vi "InsertRamp.vi"(8 "error in (no error)":errorcluster, 11 "Pulseblaster in":refnum<class "Pulseblaster.lvclass">) -> (0 "error out":errorcluster, 3 "Pulseblaster out":refnum<class "Pulseblaster.lvclass">)   [LabVIEW 2012, in "Pulseblaster.lvclass"]
uses:
  Pulseblaster.lvclass
  PulseBlaster.lvlib
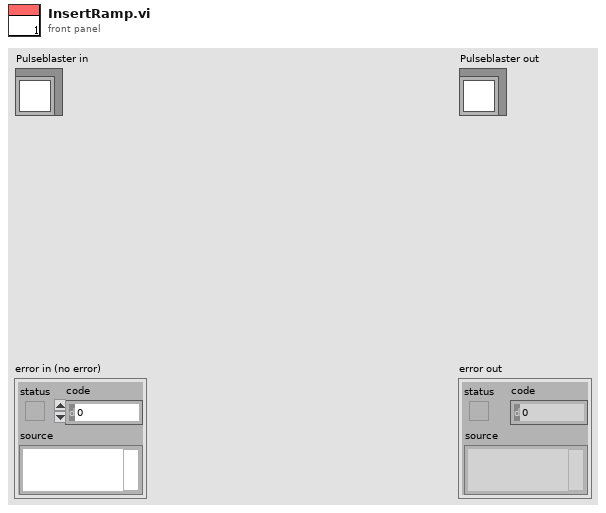
[diagram p1: front panel]
types:
  T1 = cluster{"Output Bits":u32, "Data Field":u32, "OP Code":u8, "Delay Count":u32}[]
  T2 = cluster{"Ramp Index":i32, "Ramp Time":dbl, "Number of Steps":i32}[]
  T3 = cluster{"Output Bits":u32, "Data Field":u32, "OP Code":u8, "Delay Count":u64}[]
  T4 = cluster{"Output Bits":u32, "Data Field":u32, "OP Code":u8, "Delay Count":u64}
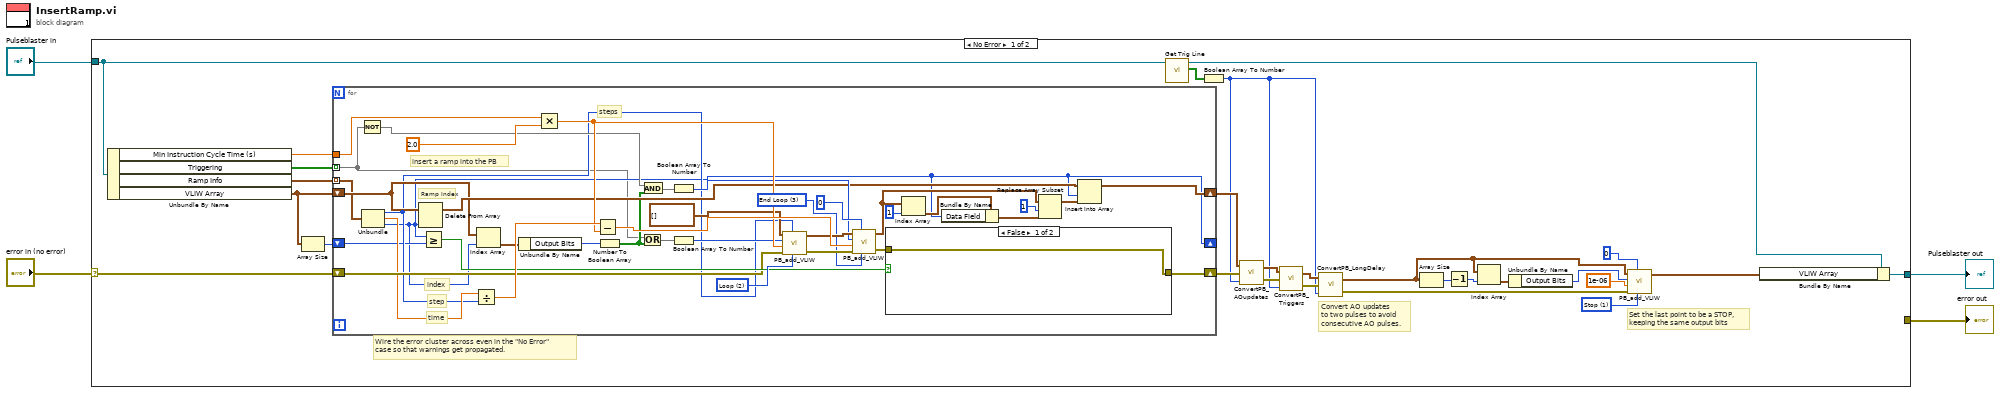
[diagram p0: block diagram]
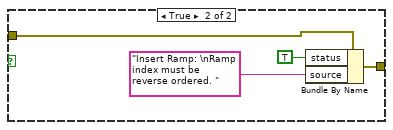
[diagram p2: hidden frame]
diagram:
  n1 = case shown="No Error" "error in (no error)" {
    selector: "error in (no error)" -> [w27 w76]
    tunnel: [_ w76] -> w3
    tunnel: [w25 w75] -> w1
    tunnel: "Pulseblaster in" -> [w26 w75]
    frame No Error {
      w14 = u8 1 items=["Continue", "Stop", "Loop", "End Loop", "Jump", "Return", "Go To", "Long Delay"] ("OP code")
      # "Convert AO updates\nto two pulses to avoid\nconsecutive AO pulses."
      # "Set the last point to be a STOP,\nkeeping the same output bits"
      # "Wire the error cluster across even in the \"No Error\"\ncase so that warnings get propagated."
      n2 = Unbundle By Name(w26) -> ("Min Instruction Cycle Time (s)"=w30:dbl, "Triggering"=w5:bool[][], "Ramp Info"=w29:T2, "VLIW Array"=w28:T3)
      n3 = Array Size(array=w28) -> (size(s)=w31:i32)
      n4 = for {
        tunnel: w29 -> [w38] mode=indexing
        shift-right: [w41] -> w11
        shift-left: w27 -> [w42]
        shift-right: [w39] -> w10
        shift-left: w28 -> [w40]
        shift-right: [w34] -> _
        shift-left: w31 -> [w35]
        tunnel: w30 -> [w33]
        tunnel: w5 -> [w32] mode=indexing
        w60 = u8 3 items=["Continue", "Stop", "Loop", "End Loop", "Jump", "Return", "Go To", "Long Delay"] ("OP code")
        w63 = u8 2 items=["Continue", "Stop", "Loop", "End Loop", "Jump", "Return", "Go To", "Long Delay"] ("OP code")
        # "steps"
        # "step"
        # "time"
        # "index"
        # "insert a ramp into the PB"
        # "Ramp Index"
        n5 = Not(x=w32) -> (.not. x?=w45:bool[])
        n6 = Unbundle(w38) -> ("Ramp Index"=w36:i32, "Ramp Time"=w37:dbl, "Number of Steps"=w34:i32)
        n7 = Delete From Array(array=w40, index=w34) -> (array with subset deleted=w49:T3)  [unwired: 1 in, 1 out]
        n8 = Greater Or Equal?(x=w34, y=w35) -> (x >= y?=w44:bool)
        n9 = Divide(x=w37, y=w36) -> (x/y=w69:dbl)
        n10 = Index Array(array=w40, index=w34) -> (element=w65:T4)
        n11 = Unbundle By Name(w65) -> ("Output Bits"=w50:u32)
        n12 = Multiply(x=w33, y=2.0) -> (x*y=w66:dbl)
        n13 = Subtract(x=w69, y=w66) -> (x-y=w68:dbl)
        n14 = Number To Boolean Array(number=w50) -> (Boolean array=w46:bool[])
        n15 = Or(x=w32, y=w46) -> (x .or. y?=w48:bool[])
        n16 = And(x=w45, y=w46) -> (x .and. y?=w47:bool[])
        n17 = Boolean Array To Number(Boolean array=w47) -> (number=w58:u32)
        n18 = Boolean Array To Number(Boolean array=w48) -> (number=w64:u32)
        n19 = call "PB_add_VLIW.vi"("VLIW Array In"=T1 [], "Data Field"=w36, "Digital Bits"=w64, "Delay"=w66, "OP code"=w63, "error in (no error)"=w42) -> ("VLIW Array Out"=w62:T3, "error out"=w61:errorcluster)  [unwired: 1 out]
        n20 = call "PB_add_VLIW.vi"("VLIW Array In"=w62, "Data Field"=u32 0, "Digital Bits"=w58, "Delay"=w68, "OP code"=w60, "error in (no error)"=w61) -> ("VLIW Array Out"=w51:T3, "error out"=w43:errorcluster)  [unwired: 1 out]
        n21 = case shown="False" w44 {
          tunnel: [w70 w72] -> w41
          tunnel: w43 -> [w70 w71]
          frame False {
          }
          frame True {
            n22 = Bundle By Name(cluster=w71, "status"=TRUE, "source"="Insert Ramp: \nRamp index must be reverse ordered. ") -> (w72:errorcluster)
          }
        }
        n23 = Index Array(array=w51, index=1 ("Index")) -> (element=w55:T4)
        n24 = Bundle By Name(cluster=w55, "Data Field"=w34) -> (w54:T4)
        n25 = Replace Array Subset(array=w51, new element=w54, index=1) -> (w52:T3)
        n26 = Insert Into Array(array=w49, index=w34, new element=w52) -> (w39:T3)
      }
      n27 = call-dynamic "Get Trig Line.vi"("Master Device in"=w26) -> ("Full Trigger Line"=w7:bool[], "Master Device out"=w8:refnum<class "Pulseblaster.lvclass">)  [unwired: 8 in, 1 out]
      n28 = Boolean Array To Number(Boolean array=w7) -> (number=w6:u32)
      n29 = call "ConvertPB_AOupdates.vi"("Full trigger mask"=w6, "error in (no error)"=w11, "PB VLIW Array in"=w10) -> ("error out"=w21:errorcluster, "PB VLIW Array out"=w20:T3)
      n30 = call "ConvertPB_Triggers.vi"("Full trigger mask"=w6, "error in (no error)"=w21, "PB VLIW Array in"=w20) -> ("error out"=w24:errorcluster, "PB VLIW Array out"=w22:T3)
      n31 = call "ConvertPB_LongDelay.vi"("Full trigger mask"=w6, "error in (no error)"=w24, "PB VLIW Array in"=w22) -> ("error out"=w12:errorcluster, "PB VLIW Array out"=w23:T3)
      n32 = Array Size(array=w23) -> (size(s)=w18:i32)
      n33 = Decrement(x=w18) -> (x-1=w17:i32)
      n34 = Index Array(array=w23, index=w17) -> (element=w16:T4)
      n35 = Unbundle By Name(w16) -> ("Output Bits"=w19:u32)
      n36 = call "PB_add_VLIW.vi"("VLIW Array In"=w23, "Data Field"=0, "Digital Bits"=w19, "Delay"=1e-06, "OP code"=w14, "error in (no error)"=w12) -> ("VLIW Array Out"=w9:T3)  [unwired: 2 out]
      n37 = Bundle By Name(cluster=w8, "VLIW Array"=w9) -> (w25:refnum<class "Pulseblaster.lvclass">)
    }
    frame Error {
    }
  }
  "error out" <- w3
  "Pulseblaster out" <- w1
